vi "Day 13 Number Logic.vi"() -> ()   [LabVIEW 2026]
panel:
  out "Sum of Divisors 2":i32
  out "List of Divisors":i32[](array[numeric])
  in  "Input Integer":i32
  out "SUM OF DIVISOR":i32
  out "Sum of Divisors":i32
  out "Array 2":i32[](array[numeric])
  in  "N 2":i32
  out "Array":i32[](array[numeric])
  in  "N":i32
  out "Is Even?":bool
  out "Solution":string
  out "Quotient":dbl
  out "Remainder":dbl
  in  "x":dbl
  # "[E] Use Quotient & Remainder to test whether a number is even."
  # "METHOD - 1 : WITH CASE STRUCTURE"
  # "proper divisors of an integer"
  # "METHOD - 2 : WITHOUT CASE STRUCTURE/ Conditional Tunnel Shortcut"
  # "proper divisors of an integer"
  # "METHOD - 3 : WITH SHIFT REGISTERS"
  # "proper divisors of an integer"
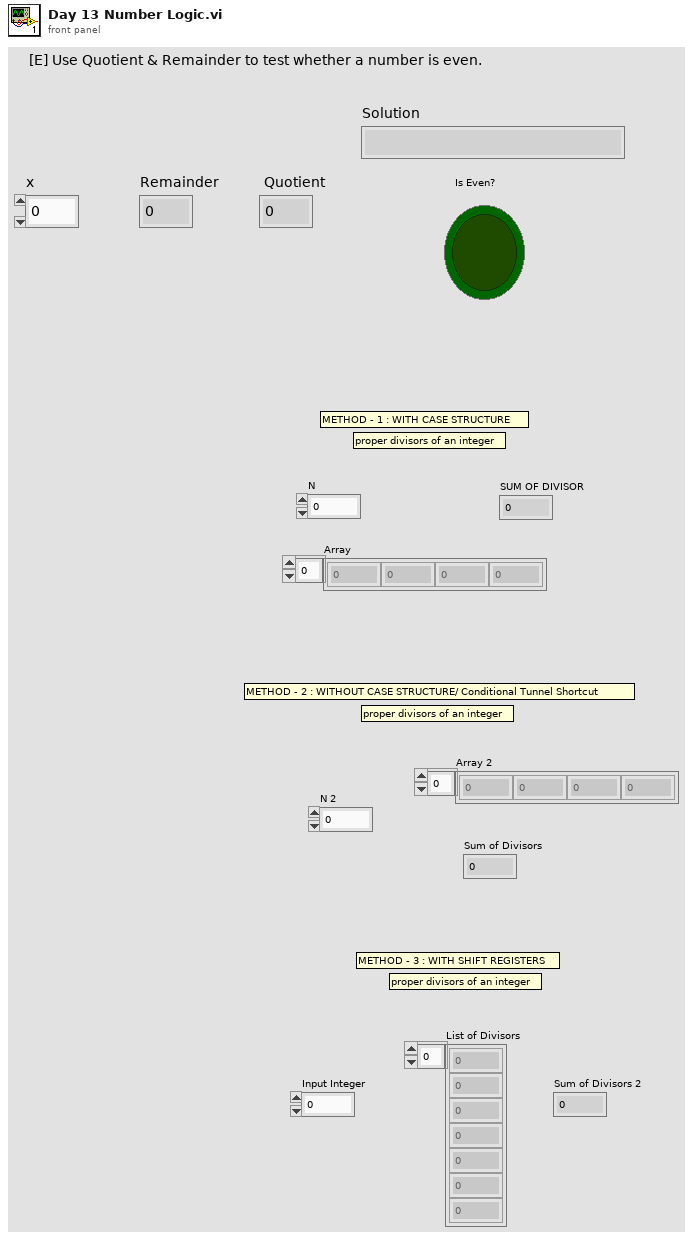
[diagram p1: front panel]
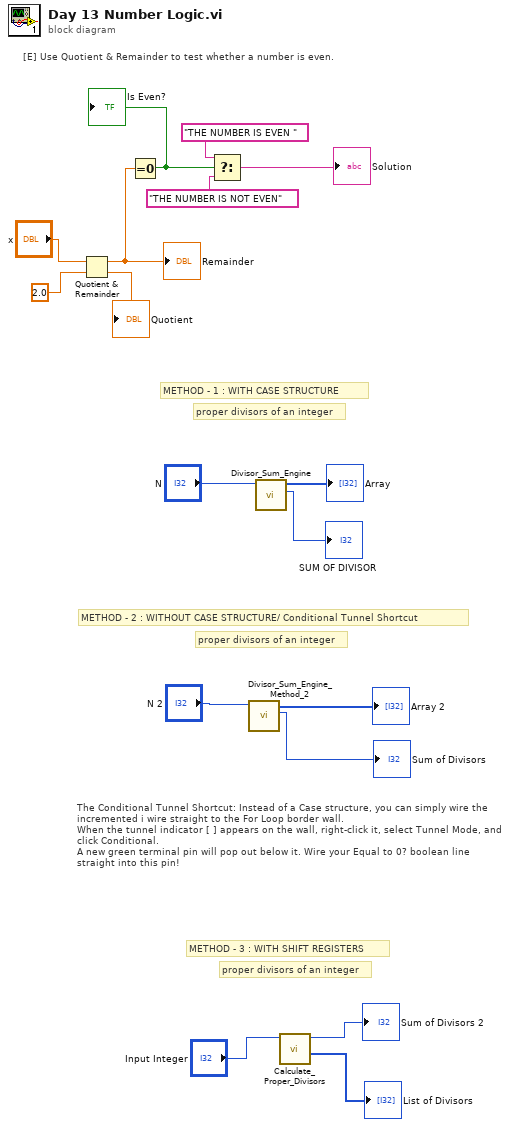
[diagram p0: block diagram]
diagram:
  # "METHOD - 3 : WITH SHIFT REGISTERS"
  # "proper divisors of an integer"
  # "The Conditional Tunnel Shortcut: Instead of a Case structure, you can simply wire the incremented i wire straight to the For Loop border wall. \nWhen the tunnel indicator [ ] appears on the wall, right-click it, select Tunnel Mode, and click Conditional. \nA new green terminal pin will pop out below it. Wire your Equal to 0? boolean line straight into this pin!"
  # "METHOD - 2 : WITHOUT CASE STRUCTURE/ Conditional Tunnel Shortcut"
  # "proper divisors of an integer"
  # "METHOD - 1 : WITH CASE STRUCTURE"
  # "proper divisors of an integer"
  # "[E] Use Quotient & Remainder to test whether a number is even."
  n1 = Quotient & Remainder(x="x", y=2.0) -> (x-y*floor(x/y)=w14:dbl, floor(x/y)=→"Quotient":dbl)
  "Remainder" <- w14
  n2 = Equal To 0?(x=w14) -> (x = 0?=w10:bool)
  "Is Even?" <- w10
  n3 = Select(t="THE NUMBER IS EVEN ", s=w10, f="THE NUMBER IS NOT EVEN") -> (s? t:f=→"Solution":string)
  n4 = call "Divisor_Sum_Engine_Method_2.vi"("N"="N 2") -> ("Numeric"=→"Sum of Divisors":i32, "Array"=→"Array 2":i32[])  [unwired: 9 in]
  n5 = call "Divisor_Sum_Engine.vi"("N"="N") -> ("Numeric"=→"SUM OF DIVISOR":i32, "Array"=→"Array":i32[])  [unwired: 9 in]
  n6 = call "Calculate_Proper_Divisors.vi"("Input Integer"="Input Integer") -> ("List of Divisors"=→"List of Divisors":i32[], "Sum of Divisors"=→"Sum of Divisors 2":i32)  [unwired: 9 in]
